vi "decodeString.vi"(8 "error in (no error)":errorcluster, 10 "ByteArray":u8[](array[numeric]) format="%.0x") -> (0 "error out":errorcluster, 1 "String":string, 2 "variant":variant, 3 "RemainingBytes":u8[](array[numeric]), 5 "Type":string)   [LabVIEW 2020, in "MsgPack.lvlib"]
uses:
  MsgPack.lvlib
  <vilib>/Utility/error.llb/Error Cluster From Error Code.vi
  <vilib>/ErrorRing/Error Ring.xnode
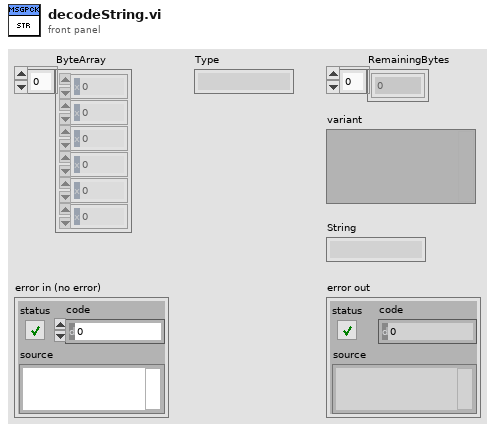
[diagram p1: front panel]
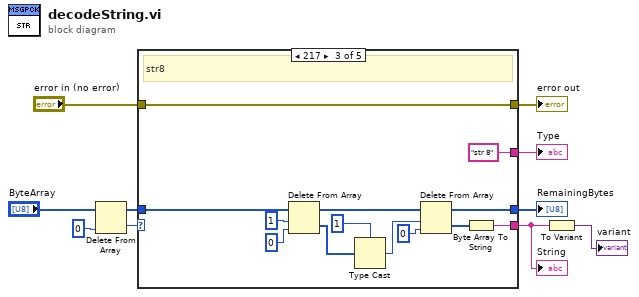
[diagram p0: block diagram]
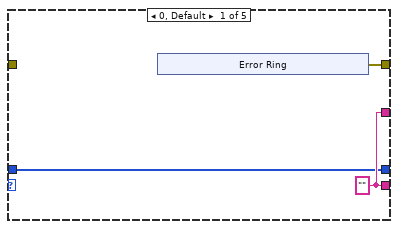
[diagram p2: hidden frame]
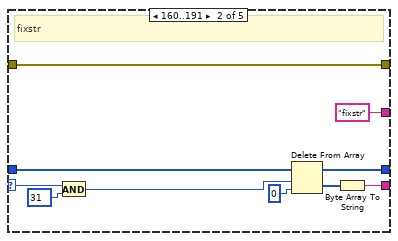
[diagram p3: hidden frame]
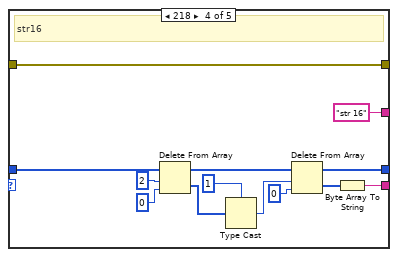
[diagram p4: hidden frame]
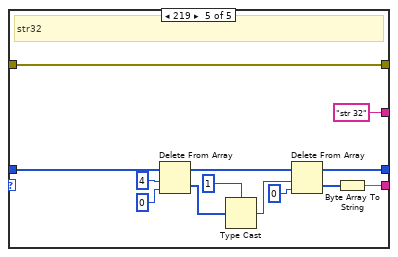
[diagram p5: hidden frame]
diagram:
  n1 = Delete From Array(array="ByteArray", index=0) -> (deleted portion=w2:u8, array with subset deleted=w4:u8[])  [unwired: 1 in]
  n2 = case shown="217" w2 {
    selector: w2 -> [_ w26 _ _ _]
    tunnel: [w13 w28 w40 w53 w66] -> w9
    tunnel: "error in (no error)" -> [_ w28 w40 w53 w66]
    tunnel: [w12 "fixstr" "str 8" "str 16" "str 32"] -> w7
    tunnel: [w12 w24 w38 w52 w65] -> w6
    tunnel: w4 -> [w11 w23 w31 w51 w59]
    tunnel: [w11 w20 w33 w44 w58] -> w3
    frame 0, Default {
      w12 = ""
      n3 = xnode "Error Ring"() -> ("error out"=w13:errorcluster)
    }
    frame 160..191 {
      # "fixstr"
      n4 = And(x=w26, y=u8 31) -> (x .and. y?=w22:u8)
      n5 = Delete From Array(array=w23, length=w22, index=0) -> (deleted portion=w21:u8[], array with subset deleted=w20:u8[])
      n6 = Byte Array To String(unsigned byte array=w21) -> (string=w24:string)
    }
    frame 217 {
      # "str8"
      n7 = Delete From Array(array=w31, length=1, index=0) -> (deleted portion=w36:u8[], array with subset deleted=w35:u8[])
      n8 = Type Cast(type=u8 1 ("index"), x=w36) -> (*(type *) &x=w34:u8)
      n9 = Delete From Array(array=w35, length=w34, index=0) -> (deleted portion=w32:u8[], array with subset deleted=w33:u8[])
      n10 = Byte Array To String(unsigned byte array=w32) -> (string=w38:string)
    }
    frame 218 {
      # "str16"
      n11 = Delete From Array(array=w51, length=2, index=0) -> (deleted portion=w48:u8[], array with subset deleted=w47:u8[])
      n12 = Type Cast(type=u16 1 ("index"), x=w48) -> (*(type *) &x=w46:u16)
      n13 = Delete From Array(array=w47, length=w46, index=0) -> (deleted portion=w45:u8[], array with subset deleted=w44:u8[])
      n14 = Byte Array To String(unsigned byte array=w45) -> (string=w52:string)
    }
    frame 219 {
      # "str32"
      n15 = Delete From Array(array=w59, length=4, index=0) -> (deleted portion=w62:u8[], array with subset deleted=w63:u8[])
      n16 = Type Cast(type=u32 1 ("index"), x=w62) -> (*(type *) &x=w64:u32)
      n17 = Delete From Array(array=w63, length=w64, index=0) -> (deleted portion=w57:u8[], array with subset deleted=w58:u8[])
      n18 = Byte Array To String(unsigned byte array=w57) -> (string=w65:string)
    }
  }
  "error out" <- w9
  "Type" <- w7
  "String" <- w6
  "RemainingBytes" <- w3
  n19 = To Variant(anything=w6) -> (Variant=→"variant":variant)
